vi "getVIinfo.vi"(11 "path":path) -> (0 "values":string[](array[string]), 1 "titles":string[](array[string]), 2 "Automatic:Error:Handling":bool, 3 "Contains:Compiled:Code":bool, 4 "Execution:State":T3(ring))   [LabVIEW 2022 SP3]
panel:
  out "VI:Total:Size":u32
  out "LabVIEW:Revision:Number":u32
  out "Number:of:subVIs":i32
  out "Execution:Priority":T1(ring)
  out "Execution:Thread":T2(ring)
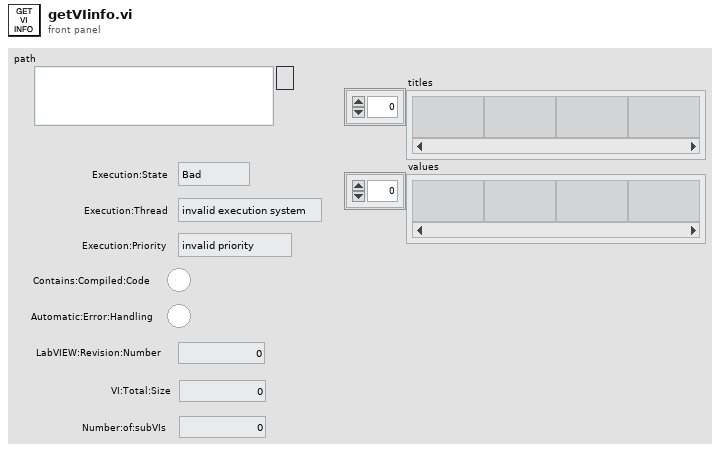
[diagram p1: front panel]
types:
  T1 = enum32{"invalid priority", "background priority", "normal priority", "above normal priority", "high priority", "time critical priority", "subroutine"}
  T2 = enum32{"invalid execution system", "user interface", "standard", "instrument i/o", "data acquisition", "other 1", "other 2", "same as caller"}
  T3 = enum32{"Bad", "Idle", "Run top level", "Running"}
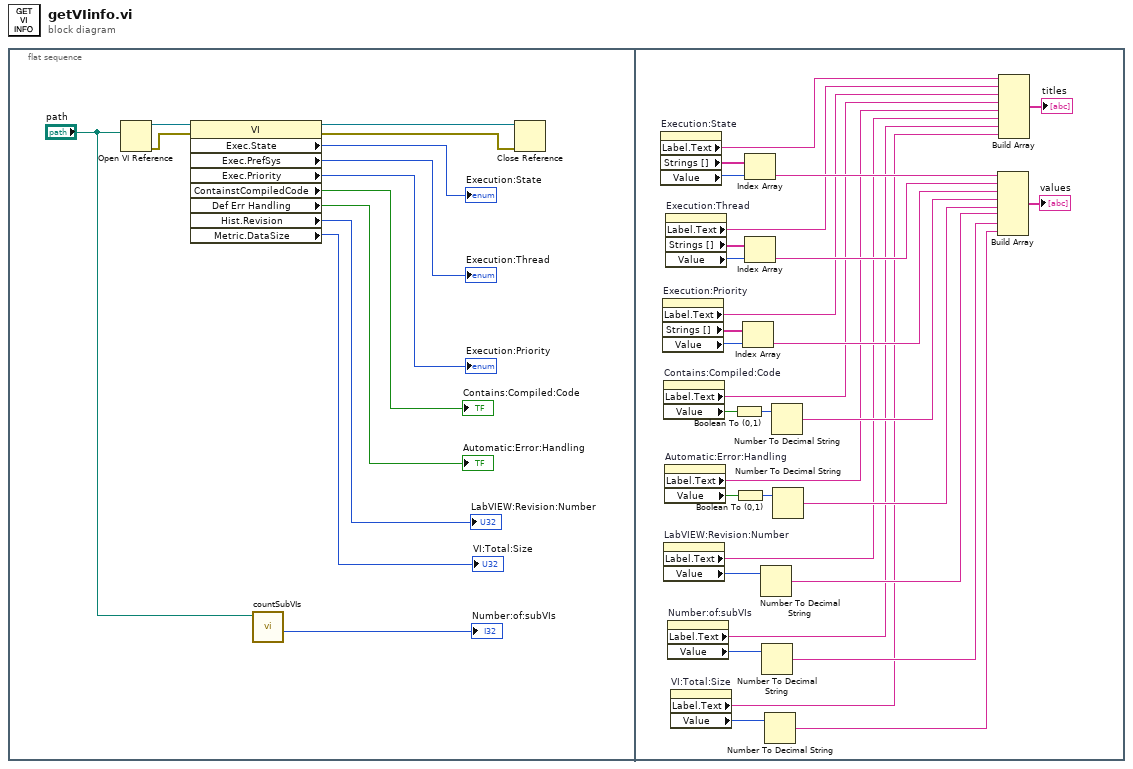
[diagram p0: block diagram]
diagram:
  n1 = flat-sequence {
    frame #0 {
      n2 = Open VI Reference(vi path="path") -> (vi reference=w10:refnum<vi>, error out=w12:errorcluster)  [unwired: 5 in]
      n3 = property class="VI"(reference=w10, error in=w12) -> (reference out=w11:refnum<vi>, error out=w13:errorcluster, "Exec.State"=→"Execution:State":T3, "Exec.PrefSys"=→"Execution:Thread":T2, "Exec.Priority"=→"Execution:Priority":T1, "ContainstCompiledCode"=→"Contains:Compiled:Code":bool, "Def Err Handling"=→"Automatic:Error:Handling":bool, "Hist.Revision"=→"LabVIEW:Revision:Number":u32, "Metric.DataSize"=→"VI:Total:Size":u32)
      n4 = call "countSubVIs.vi"("vi path"="path") -> ("nSubVIs"=→"Number:of:subVIs":i32)  [unwired: 9 in, 1 out]
      n5 = Close Reference(reference=w11, error in (no error)=w13) -> ()  [unwired: 1 out]
    }
    frame #1 {
      n6 = property on="Execution:State" class="Enum (strict)"() -> ("Label.Text"=w20:string, "Strings []"=w17:string[], "Value"=w33:T3)  [unwired: 2 in, 2 out]
      n7 = property on="Execution:Priority" class="Enum (strict)"() -> ("Label.Text"=w22:string, "Strings []"=w19:string[], "Value"=w35:T1)  [unwired: 2 in, 2 out]
      n8 = property on="Contains:Compiled:Code" class="Bool (strict)"() -> ("Label.Text"=w23:string, "Value"=w27:bool)  [unwired: 2 in, 2 out]
      n9 = property on="LabVIEW:Revision:Number" class="DigNum (strict)"() -> ("Label.Text"=w25:string, "Value"=w30:u32)  [unwired: 2 in, 2 out]
      n10 = property on="Automatic:Error:Handling" class="Bool (strict)"() -> ("Label.Text"=w24:string, "Value"=w32:bool)  [unwired: 2 in, 2 out]
      n11 = property on="Execution:Thread" class="Enum (strict)"() -> ("Label.Text"=w21:string, "Strings []"=w18:string[], "Value"=w34:T2)  [unwired: 2 in, 2 out]
      n12 = property on="Number:of:subVIs" class="DigNum (strict)"() -> ("Label.Text"=w26:string, "Value"=w29:i32)  [unwired: 2 in, 2 out]
      n13 = property on="VI:Total:Size" class="DigNum (strict)"() -> ("Label.Text"=w15:string, "Value"=w16:u32)  [unwired: 2 in, 2 out]
      n14 = Boolean To (0,1)(Boolean=w27) -> (0, 1=w28:i16)
      n15 = Boolean To (0,1)(Boolean=w32) -> (0, 1=w31:i16)
      n16 = Index Array(array=w19, index=w35) -> (element=w38:string)
      n17 = Index Array(array=w17, index=w33) -> (element=w36:string)
      n18 = Index Array(array=w18, index=w34) -> (element=w37:string)
      n19 = Number To Decimal String(number=w30) -> (decimal integer string=w41:string)  [unwired: 1 in]
      n20 = Number To Decimal String(number=w29) -> (decimal integer string=w42:string)  [unwired: 1 in]
      n21 = Number To Decimal String(number=w16) -> (decimal integer string=w14:string)  [unwired: 1 in]
      n22 = Number To Decimal String(number=w28) -> (decimal integer string=w39:string)  [unwired: 1 in]
      n23 = Number To Decimal String(number=w31) -> (decimal integer string=w40:string)  [unwired: 1 in]
      n24 = Build Array(w36, w37, w38, w39, w40, w41, w42, w14) -> (→"values":string[])
      n25 = Build Array(w20, w21, w22, w23, w24, w25, w26, w15) -> (→"titles":string[])
    }
  }
